vi "EXDIR-YAML_Inefficient_YAML_to_Tree-like_Dictionary.vi"() -> ()   [LabVIEW 2016]
panel:
  out "items":cluster{"key":variant, "value":variant}[](array[cluster])
  out "array":string[](array[string])
  out "YAML in raw":string
  in  "YAML in":string
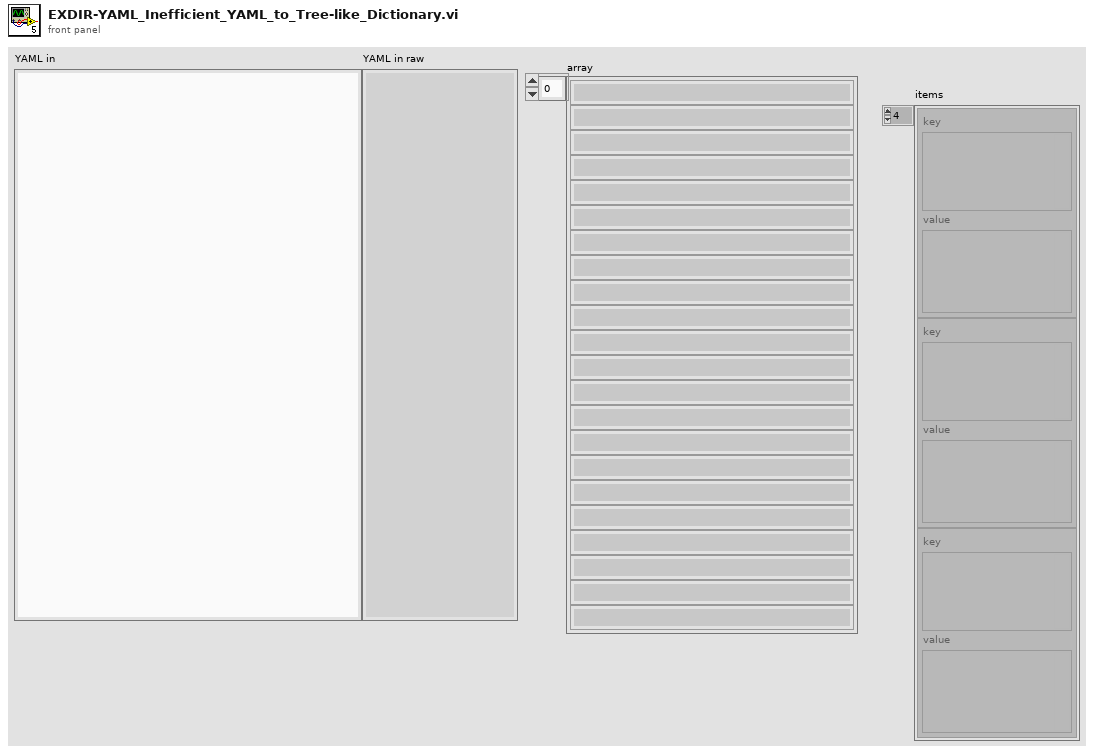
[diagram p1: front panel]
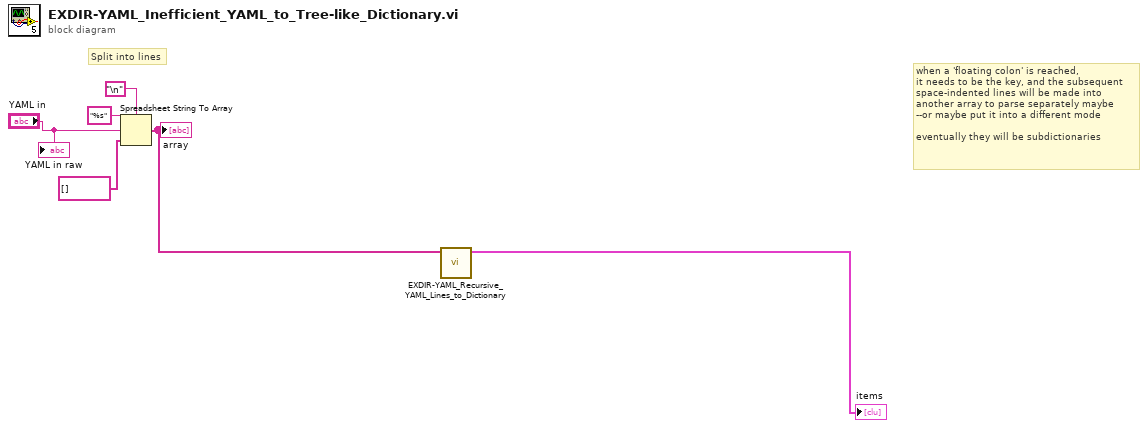
[diagram p0: block diagram]
diagram:
  # "when a 'floating colon' is reached,\nit needs to be the key, and the subsequent\nspace-indented lines will be made into \nanother array to parse separately maybe\n--or maybe put it into a different mode\n\neventually they will be subdictionaries"
  # "Split into lines"
  n1 = Spreadsheet String To Array(delimiter (Tab)="\n", format string="%s", spreadsheet string="YAML in", array type (2D Dbl)=string[] []) -> (array=w2:string[])
  "array" <- w2
  n2 = call "EXDIR-YAML_Recursive_YAML_Lines_to_Dictionary.vi"("Array of YAML Lines"=w2) -> ("Dictionary Items"=→"items":cluster{"key":variant, "value":variant}[])  [unwired: 9 in, 1 out]
  "YAML in raw" <- "YAML in"
